vi "DBCreateTable-Log.vi"(7 "Drop?":bool, 8 "error in (no error)":errorcluster, 11 "ProcessState in":T1) -> (0 "error out":errorcluster, 3 "ProcessState out":T1)   [LabVIEW 2015, in "CopyUtility.lvlib"]
uses:
  CopyUtility.lvlib
  controls/ProcessState.ctl
  <vilib>/drjdpowell/SQLite Library/SQL Connection/Connection.lvclass
  DBToolkit/DBToolkit.lvlib
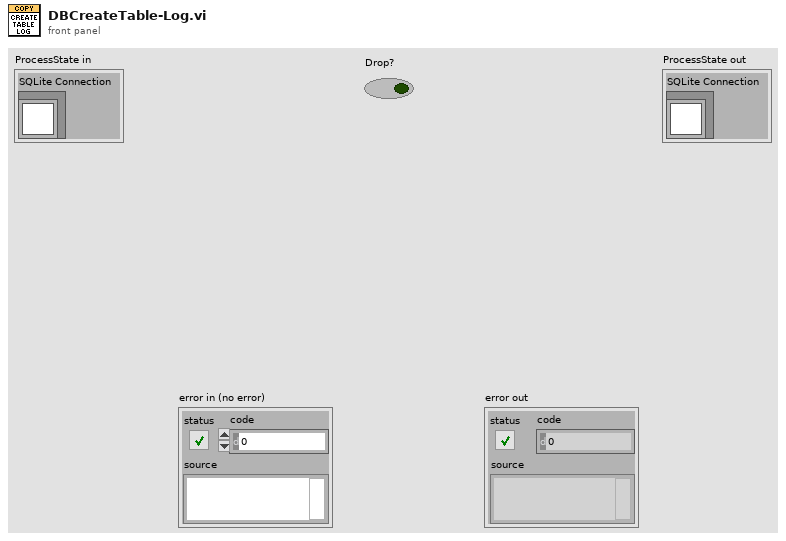
[diagram p1: front panel]
types:
  T1 = typedef "CopyUtility.lvlib/ProcessState.ctl" = cluster{"SQLite Connection":refnum<class "Connection.lvclass">}
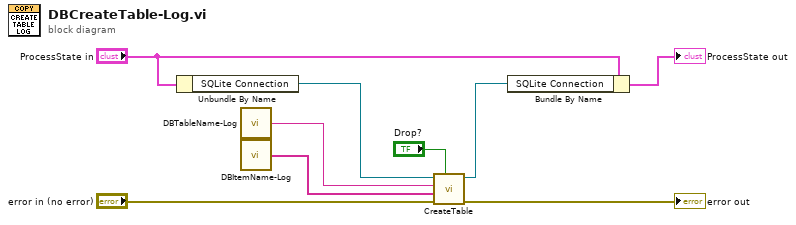
[diagram p0: block diagram]
diagram:
  n1 = Unbundle By Name("ProcessState in") -> ("SQLite Connection"=w5:refnum<class "Connection.lvclass">)
  n2 = call "DBTableName-Log.vi"() -> ("DB Table Name"=w3:string)  [unwired: 5 in]
  n3 = call "DBItemName-Log.vi"() -> ("Items"=w2:string[])  [unwired: 5 in]
  n4 = call "CreateTable.vi"("Drop?"="Drop?", "error in (no error)"="error in (no error)", "Items"=w2, "Table Name"=w3, "SQLite Connection in"=w5) -> ("error out"=→"error out":errorcluster, "SQLite Connection out"=w4:refnum<class "Connection.lvclass">)  [unwired: 5 in]
  n5 = Bundle By Name(cluster="ProcessState in", "SQLite Connection"=w4) -> (→"ProcessState out":T1)
